vi "Unflatten to PDU1.vi"(8 "error in (no error)":errorcluster, 10 "Modbus data unit data":u8[](array[numeric])) -> (0 "error out":errorcluster, 3 "Modbus data unit out":T1={"function"=1, "Data"=[]} {"function" items=["Read Discrete Inputs"=2, "Read Coils"=1, "Write Single Coil"=5, "Write Multiple Coils"=15, "Read Input Register"=4, "Read Holding Registers"=3, "Write Single Register"=6, "Write Multiple Registers"=16, "Read/Write Multiple Registers"=23, "Mask Write Register"=22, "Read FIFO Queue"=24, "Read File Record"=20, "Write File Record"=21, "Read Exception Status"=7, "Diagnostic"=8, "Get Com Event Counter"=11, "Get Com Event Log"=12, "Report Slave ID"=17, "Read Device Identification"=43]; "Data" format="%.0x"})   [LabVIEW 2019, in "NI_modbus_upd.lvlib"]
uses:
  NI_modbus_upd.lvlib
  Ctl/MB Modbus Data Unit.ctl
  Function.ctl
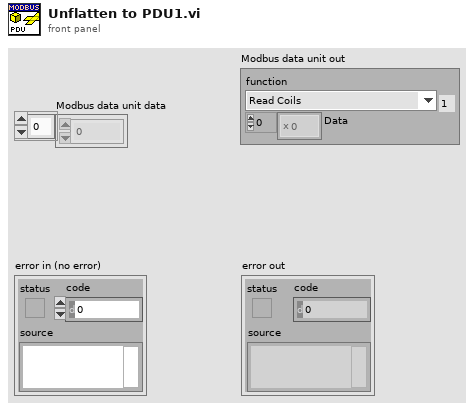
[diagram p1: front panel]
types:
  T1 = typedef "NI_modbus_upd.lvlib/MB Modbus Data Unit.ctl" = cluster{"function":T2, "Data":u8[]}
  T2 = typedef "NI_modbus_upd.lvlib/Function.ctl" = u8
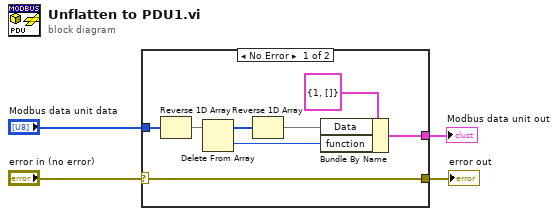
[diagram p0: block diagram]
diagram:
  n1 = case shown="No Error" "error in (no error)" {
    selector: "error in (no error)" -> [w5 w13]
    tunnel: [w12 _] -> w4
    tunnel: "Modbus data unit data" -> [w9 _]
    tunnel: [w5 w13] -> w1
    frame No Error {
      n2 = Reverse 1D Array(array=w9) -> (reversed array=w8:u8[])
      n3 = Delete From Array(array=w8) -> (deleted portion=w10:u8, array with subset deleted=w6:u8[])  [unwired: 2 in]
      n4 = Reverse 1D Array(array=w6) -> (reversed array=w7:u8[])
      n5 = Bundle By Name(cluster=T1 {"function"=1, "Data"=[]} ("modbus data unit"), "Data"=w7, "function"=w10) -> (w12:T1)
    }
    frame Error {
    }
  }
  "error out" <- w1
  "Modbus data unit out" <- w4
